vi "Network_ApplyDHCP.vi"(7 "DevInfo Original":T1={"Hostname"="", "IPAddress"="", "MAC"="", "SerialNum"="", "Model"="", "Status"="", "FW"="", "OSDesc"="", "ImgTitle"="", "ImgDesc"="", "ImgVer"="", "ImgID"="", "IP Address Request Mode"=1, "SubnetMask"="", "Gateway"="", "DNSServer"=""} {"IP Address Request Mode" items=["Static"=1, "DHCP/Link-Local"=2, "Link-Local Only"=4, "DHCP Only"=8]}, 8 "error in (no error)":errorcluster, 11 "DevInfo Modified":T1={"Hostname"="", "IPAddress"="", "MAC"="", "SerialNum"="", "Model"="", "Status"="", "FW"="", "OSDesc"="", "ImgTitle"="", "ImgDesc"="", "ImgVer"="", "ImgID"="", "IP Address Request Mode"=1, "SubnetMask"="", "Gateway"="", "DNSServer"=""} {"IP Address Request Mode" items=["Static"=1, "DHCP/Link-Local"=2, "Link-Local Only"=4, "DHCP Only"=8]}) -> (0 "error out":errorcluster)   [LabVIEW 2021]
uses:
  TypeDefs/DevInfo.ctl
  TypeDefs/TargetAccess.ctl
  <vilib>/nisyscfg/Save Changes (System).vi
  <vilib>/nisyscfg/Close (System).vi
  <resource>/objmgr/nisysapi.rc
  <vilib>/nisyscfg/nisyscfg.lvlib
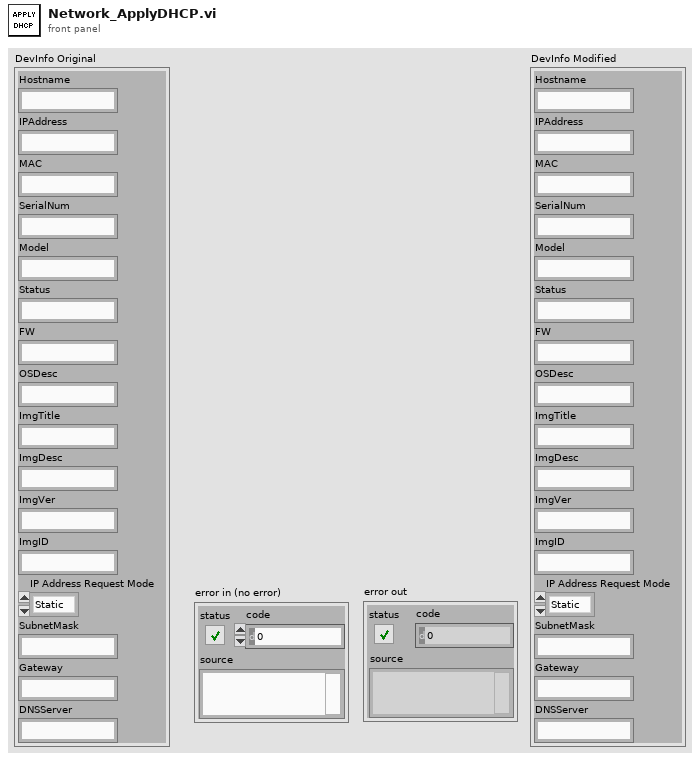
[diagram p1: front panel]
types:
  T1 = typedef "DevInfo.ctl" = cluster{"Hostname":string, "IPAddress":string, "MAC":string, "SerialNum":string, "Model":string, "Status":string, "FW":string, "OSDesc":string, "ImgTitle":string, "ImgDesc":string, "ImgVer":string, "ImgID":string, "IP Address Request Mode":i32, "SubnetMask":string, "Gateway":string, "DNSServer":string}
  T2 = typedef "TargetAccess.ctl" = enum16{"Read-Only", "Admin"}
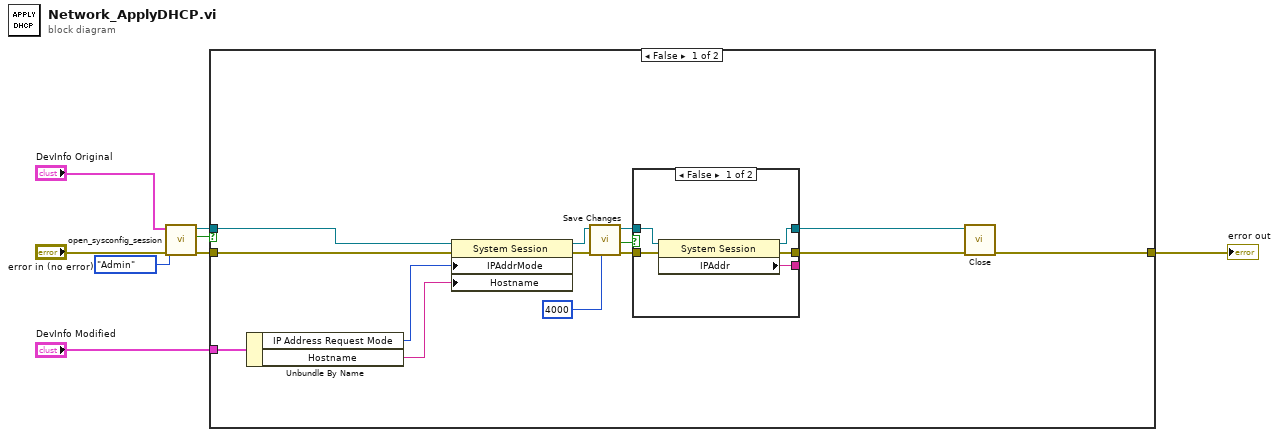
[diagram p0: block diagram]
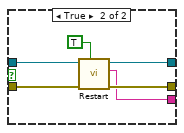
[diagram p2: hidden frame]
diagram:
  n1 = call "open_sysconfig_session.vi"("error in (no error)"="error in (no error)", "Target Access"=TargetAccess."Admin", "DevInfo"="DevInfo Original") -> ("error out"=w5:errorcluster, "Cancelled"=w6:bool, "Session Out"=w4:refnum<k21>)  [unwired: 6 in]
  n2 = case shown="False" w6 {
    tunnel: w5 -> [w15 w34]
    tunnel: w4 -> [w17 _]
    tunnel: "DevInfo Modified" -> [w16 _]
    tunnel: [w9 w34] -> w2
    frame False {
      n3 = Unbundle By Name(w16) -> ("IP Address Request Mode"=w11:i32, "Hostname"=w10:string)
      n4 = property class="System Session"(reference=w17, error in=w15, "IPAddrMode"=w11, "Hostname"=w10) -> (reference out=w18:refnum<k21>, error out=w19:errorcluster)
      n5 = call-poly <vilib>:"Save Changes.vi"("Remote Timeout (300,000 ms)"=u32 4000, "error in (no error)"=w19, "Session in"=w18) -> ("error out"=w21:errorcluster, "Changes Require Restart"=w20:bool, "Session out"=w22:refnum<k21>)  [unwired: 5 in, 1 out]
      n6 = case shown="False" w20 {
        tunnel: w21 -> [w27 w33]
        tunnel: [w26 w32] -> w13
        tunnel: w22 -> [w25 w31]
        tunnel: [w24 w30] -> w14
        tunnel: [w23 w28] -> _
        frame False {
          n7 = property class="System Session"(reference=w25, error in=w27) -> (reference out=w24:refnum<k21>, error out=w26:errorcluster, "IPAddr"=w23:string)
        }
        frame True {
          n8 = call <vilib>:"Restart.vi"("Wait Until Complete (T)"=TRUE ("wait until complete (T)"), "error in (no error)"=w33, "Session in"=w31) -> ("error out"=w32:errorcluster, "New IP Address"=w28:string, "Session out"=w30:refnum<k21>)  [unwired: 6 in]
        }
      }
      n9 = call-poly <vilib>:"Close.vi"("error in (no error)"=w13, "Session in"=w14) -> ("error out"=w9:errorcluster)  [unwired: 9 in]
    }
    frame True {
    }
  }
  "error out" <- w2
